vi "4-1mux_int.vi"(4 "Select(LSB)":bool, 6 "Select(MSB)":bool, 8 "Input4":dbl, 9 "Input3":dbl, 10 "Input2":dbl, 11 "Input1":dbl) -> (2 "Numeric 5":dbl)   [LabVIEW 2011]
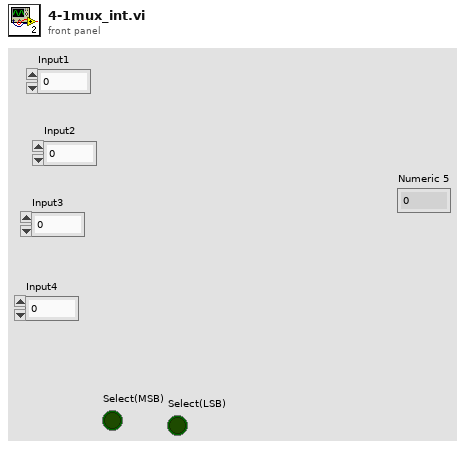
[diagram p1: front panel]
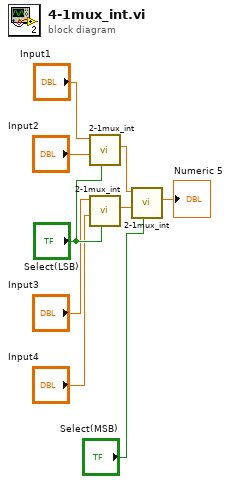
[diagram p0: block diagram]
diagram:
  n1 = call "2-1mux_int.vi"("Select"="Select(LSB)", "Input2"="Input2", "Input1"="Input1") -> ("Output"=w4:dbl)  [unwired: 8 in]
  n2 = call "2-1mux_int.vi"("Select"="Select(LSB)", "Input2"="Input4", "Input1"="Input3") -> ("Output"=w3:dbl)  [unwired: 8 in]
  n3 = call "2-1mux_int.vi"("Select"="Select(MSB)", "Input2"=w3, "Input1"=w4) -> ("Output"=→"Numeric 5":dbl)  [unwired: 8 in]
